vi "Continuous UI update loop.vi"() -> ()   [LabVIEW 2013]
uses:
  Typedefs/Read Write Enum.ctl
  Global Variables/gl_UI Ctrl Refs.vi
  Global Variables/General Globals.vi
panel:
  out "Logging queue (ind)":i32 caption="Elements accumulating\nin the logging queue"
  out "AOL Z-stack Chirps Ready (ind)":bool
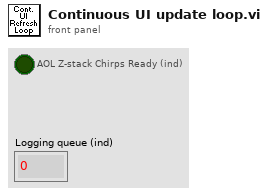
[diagram p1: front panel]
types:
  T1 = typedef "UI ctrl refs cluster.ctl" = cluster{"Top level VI path":path, "Top level VI ref":refnum<vi>, "User menu ref":refnum<k9>, "Sub Panel control":refnum<vi>, "Imaging Param Tab":refnum<vi>, "Occurrence-Start drivers":refnum<k4>, "Occurrence-Speed logging initialised":refnum<k4>, "Occurrence-XYZ stage initialised":refnum<k4>, "Exit button":refnum<vi>, "Status ind":refnum<vi>, "Return to Origin":refnum<vi>, "Speed Logging":refnum<vi>, "Time Lapse":refnum<vi>, "Live Imaging":refnum<vi>, "AOL Z Stack":refnum<vi>, "Motor Z Stack":refnum<vi>, "Funct Acq button":refnum<vi>, "Hard Shutter":refnum<vi>, "Virtual Shutter":refnum<vi>, "Laser Power":refnum<vi>, "AOL Mode":refnum<vi>, "Frame Size":refnum<vi>, "Field of View":refnum<vi>, "Dwell Time":refnum<vi>, "Zoom":refnum<vi>, "AOL Z":refnum<vi>, "Objective":refnum<vi>, "Axis":refnum<vi>, "Paths & Names":refnum<vi>, "Experiment folder path (ind.)":refnum<vi>, "Last State (Ind.)":refnum<vi>, "Laser wavelength ind (nm)":refnum<vi>, "Averages":refnum<vi>, "Angle (degrees)":refnum<vi>, "X centre":refnum<vi>, "Y centre":refnum<vi>, "Plane Mode":refnum<vi>, "# Planes":refnum<vi>, "Z Start":refnum<vi>, "Z Stop":refnum<vi>, "Z Step":refnum<vi>, "PMT 1":refnum<vi>, "PMT 2":refnum<vi>, "Stage XYZ Position":refnum<vi>, "Pockels@Z Start":refnum<vi>, "Pockels@Z Stop":refnum<vi>, "Obtain Z Start":refnum<vi>, "Obtain Z Stop":refnum<vi>, "Live stim.trig.period":refnum<vi>, "Live stim.trig.enable":refnum<vi>, "Funct. Acq. Pockels Modulation":refnum<vi>, "Enable Video Recording":refnum<vi>, "Video Record-Live Imaging":refnum<vi>, "Video Record-Funct acq":refnum<vi>, "AOL Z-stack Chirps Ready (ind)":refnum<vi>, "Center freq ind (nm)":refnum<vi>, "Logging queue (ind)":refnum<vi>, "Back aperture power (ind.)":refnum<vi>, "Power after objective (ind.)":refnum<vi>, "Switch user":refnum<vi>}
  T2 = typedef "Read Write Enum.ctl" = enum16{"Read", "Write"}
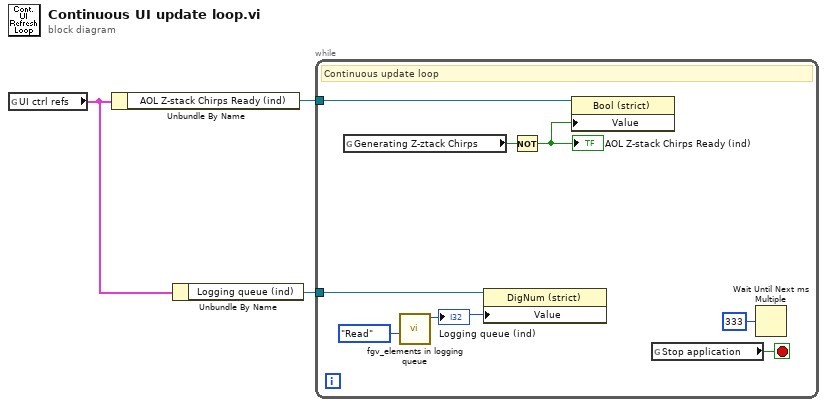
[diagram p0: block diagram]
diagram:
  n1 = global read "gl_UI Ctrl Refs.vi" "UI ctrl refs"() -> (w2:T1)
  n2 = Unbundle By Name(w2) -> ("AOL Z-stack Chirps Ready (ind)"=w3:refnum<vi>)
  n3 = Unbundle By Name(w2) -> ("Logging queue (ind)"=w1:refnum<vi>)
  n4 = while {
    tunnel: w3 -> [w6]
    tunnel: w1 -> [w4]
    stop <- w9 stop-if-true
    # "Continuous update loop"
    n5 = global read "General Globals.vi" "Generating Z-ztack Chirps"() -> (w11:bool)
    n6 = call "fgv_elements in logging queue.vi"("Function"=Read_Write_Enum."Read") -> ("Elements in logging queue"=w5:i32)  [unwired: 9 in, 1 out]
    "Logging queue (ind)" <- w5
    n7 = property class="DigNum (strict)"(reference=w4, "Value"=w5) -> ()  [unwired: 1 in, 2 out]
    n8 = Not(x=w11) -> (.not. x?=w7:bool)
    "AOL Z-stack Chirps Ready (ind)" <- w7
    n9 = property class="Bool (strict)"(reference=w6, "Value"=w7) -> ()  [unwired: 1 in, 2 out]
    n10 = global read "General Globals.vi" "Stop application"() -> (w9:bool)
    n11 = Wait Until Next ms Multiple(millisecond multiple=u32 333) -> ()  [unwired: 1 out]
  }
